vi "Chi-Squared (Non-Central) Random.vi"(6 "seed":i32=-1, 7 "reset":bool, 9 "d":dbl, 10 "k":i32=1, 11 "samples":i32=128) -> (0 "error":i32, 3 "chi-squared(nc) random data":dbl[](array[numeric]))   [LabVIEW 2020, in "NI_Gmath.lvlib"]
doc: "Generates random values from a variate X, where X describes the selected distribution type. You must manually select the polymorphic instance to use."
uses:
  <vilib>/gmath/NI_Gmath.lvlib
panel:
  # "Chi-Squared (Non-Central) Random"
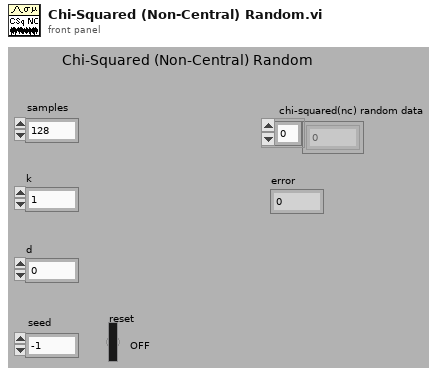
[diagram p1: front panel]
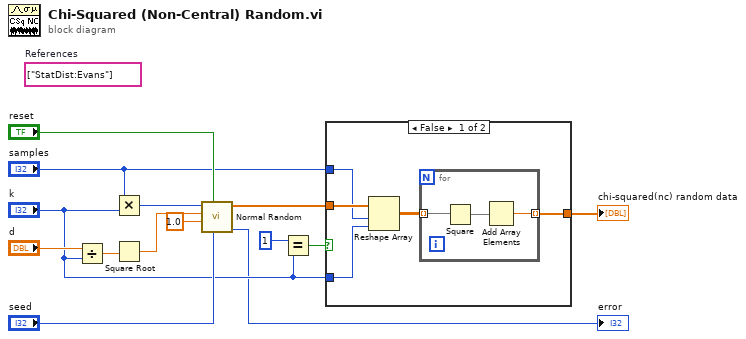
[diagram p0: block diagram]
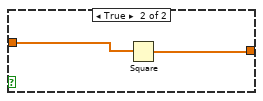
[diagram p2: hidden frame]
diagram:
  (unwired) string[] ["StatDist:Evans"]  # References
  n1 = Divide(x="d", y="k") -> (x/y=w11:dbl)
  n2 = Multiply(x="samples", y="k") -> (x*y=w8:i32)
  n3 = Square Root(x=w11) -> (sqrt(x)=w10:dbl)
  n4 = call <vilib>:"Normal Random.vi"("seed"="seed", "reset"="reset", "std"=1.0, "mean"=w10, "samples"=w8) -> ("error"=→"error":i32, "normal random data"=w4:dbl[])  [unwired: 5 in]
  n5 = Equal?(x=1, y="k") -> (x = y?=w6:bool)
  n6 = case shown="False" w6 {
    tunnel: "k" -> [w16 _]
    tunnel: w4 -> [w18 w23]
    tunnel: "samples" -> [w17 _]
    tunnel: [w15 w24] -> w2
    frame False {
      n7 = Reshape Array(w18, w17, w16) -> (w19:dbl[][])
      n8 = for {
        tunnel: w19 -> [w22] mode=indexing
        tunnel: [w20] -> w15 mode=indexing
        n9 = Square(x=w22) -> (x^2=w21:dbl[])
        n10 = Add Array Elements(numeric array=w21) -> (sum=w20:dbl)
      }
    }
    frame True {
      n11 = Square(x=w23) -> (x^2=w24:dbl[])
    }
  }
  "chi-squared(nc) random data" <- w2
